vi "MathCad_Matrix_Set_2D.vi"(3 "error in":errorcluster, 4 "2D Array":dbl[][](array[numeric]) format="%.2f", 5 "Mathcad.IMatrixValue Refnum in":refnum<k7>, 6 "Worksheet Reference In":refnum<k7>) -> (0 "error out":errorcluster, 1 "Mathcad.IMatrixValue Refnum out":refnum<k7>, 2 "Worksheet Reference Out":refnum<k7>)   [LabVIEW 2015]
doc: "Sets the value of the reference. This must be done before inserting into a worksheet."
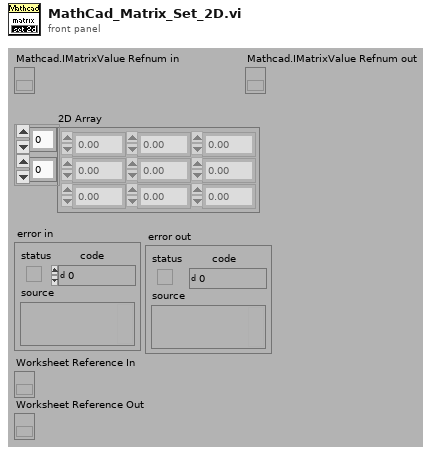
[diagram p1: front panel]
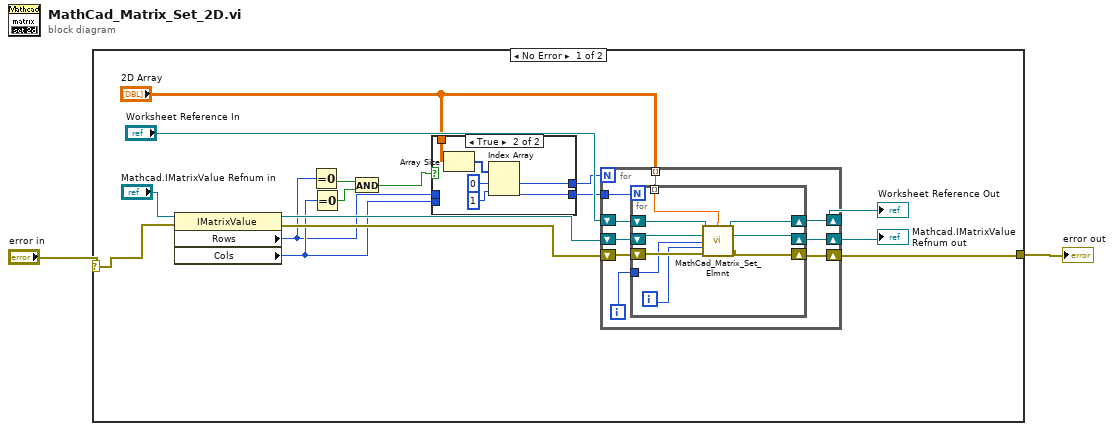
[diagram p0: block diagram]
diagram:
  n1 = case shown="No Error" "error in" {
    selector: "error in" -> [w13 w45]
    tunnel: [w18 w45] -> w1
    frame No Error {
      n2 = property class="IMatrixValue"(reference="Mathcad.IMatrixValue Refnum in", error in=w13) -> (reference out=w11:refnum<k7>, error out=w12:errorcluster, "Rows"=w4:i32, "Cols"=w6:i32)
      n3 = Equal To 0?(x=w4) -> (x = 0?=w9:bool)
      n4 = Equal To 0?(x=w6) -> (x = 0?=w8:bool)
      n5 = And(x=w9, y=w8) -> (x .and. y?=w7:bool)
      n6 = case shown="True" w7 {
        tunnel: "2D Array" -> [_ w26]
        tunnel: w6 -> [w20 _]
        tunnel: [w20 w23] -> w5
        tunnel: w4 -> [w19 _]
        tunnel: [w19 w24] -> w3
        frame False {
        }
        frame True {
          n7 = Array Size(array=w26) -> (size(s)=w25:i32[])
          n8 = Index Array(array=w25, index #1=0 ("index"), index #2=1 ("index")) -> (element #1=w24:i32, element #2=w23:i32)
        }
      }
      n9 = for {
        N: w3 -> [_]
        tunnel: "2D Array" -> [w35] mode=indexing
        shift-right: [w34] -> w18
        shift-left: w12 -> [w29]
        shift-right: [w33] -> w17
        shift-left: w11 -> [w27]
        shift-right: [w31] -> w15
        shift-left: "Worksheet Reference In" -> [w30]
        tunnel: w5 -> [w28]
        i -> [w32]
        n10 = for {
          N: w28 -> [_]
          shift-right: [w44] -> w33
          shift-left: w27 -> [w43]
          shift-right: [w42] -> w34
          shift-left: w29 -> [w41]
          tunnel: w35 -> [w40] mode=indexing
          tunnel: w32 -> [w38]
          shift-right: [w37] -> w31
          shift-left: w30 -> [w36]
          i -> [w39]
          n11 = call "MathCad_Matrix_Set_Elmnt.vi"("Worksheet Reference In"=w36, "value"=w40, "Mathcad.IMatrixValue"=w43, "row"=w38, "col"=w39, "error in"=w41) -> ("Worksheet Reference Out"=w37:refnum<k7>, "Mathcad.IMatrixValue Refnum out"=w44:refnum<k7>, "error out"=w42:errorcluster)  [unwired: 7 in]
        }
      }
      "Mathcad.IMatrixValue Refnum out" <- w17
      "Worksheet Reference Out" <- w15
    }
    frame Error {
    }
  }
  "error out" <- w1
